vi "SimpelStrategie(SubVI).vi"(4 "toggle":bool, 5 "NextTurn":dbl, 6 "BoolArray":bool[][](array[boolean]), 7 "Array":dbl[][](array[numeric])) -> (0 "toggle 2":bool, 1 "Array 3":bool[][](array[boolean]), 2 "Array 2":u8[][](array[numeric]))   [LabVIEW 2017]
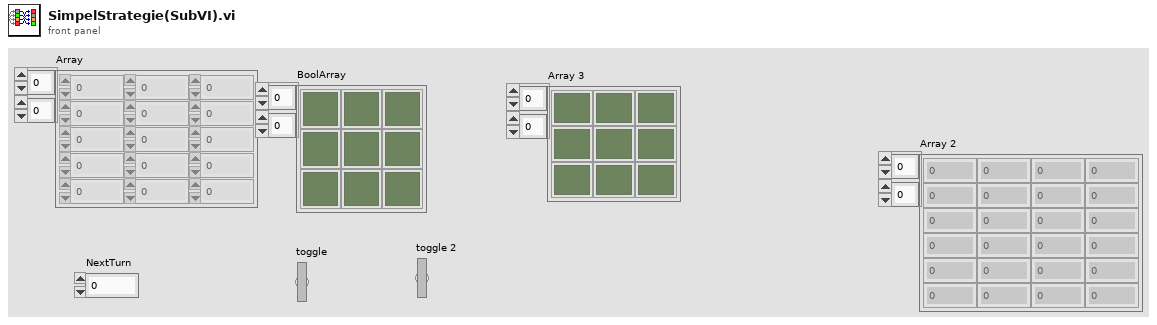
[diagram p1: front panel]
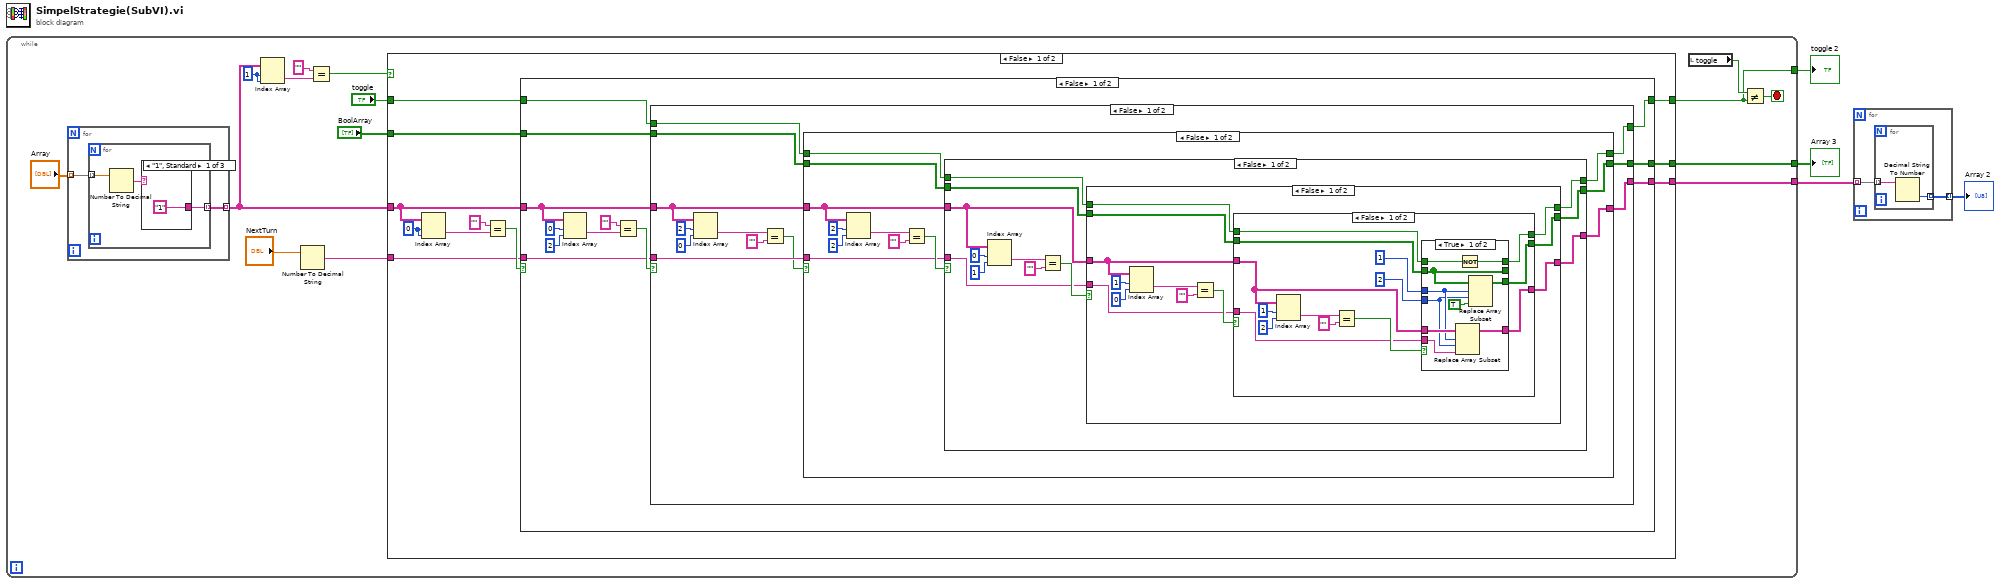
[diagram p0: block diagram]
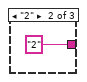
[diagram p2: hidden frame]
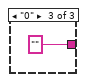
[diagram p3: hidden frame]
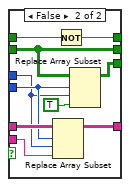
[diagram p4: hidden frame]
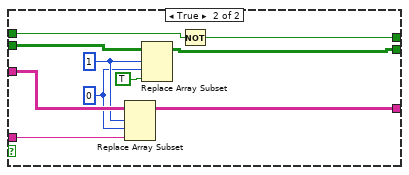
[diagram p5: hidden frame]
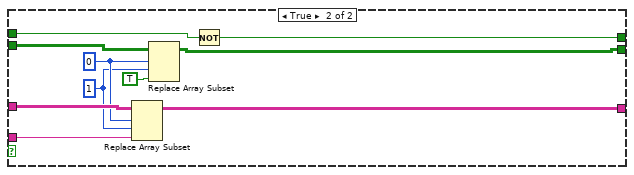
[diagram p6: hidden frame]
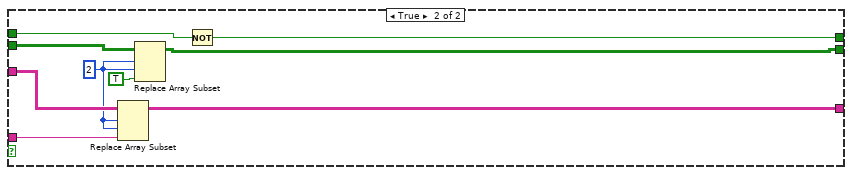
[diagram p7: hidden frame]
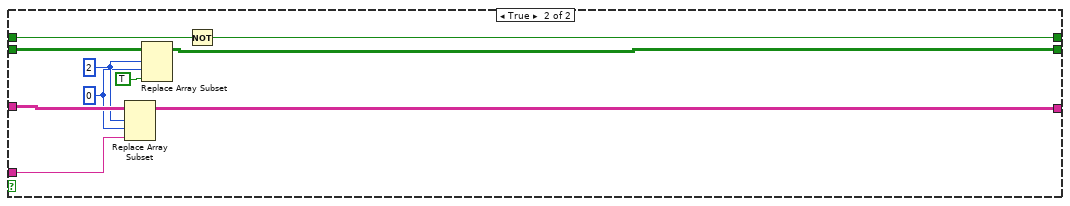
[diagram p8: hidden frame]
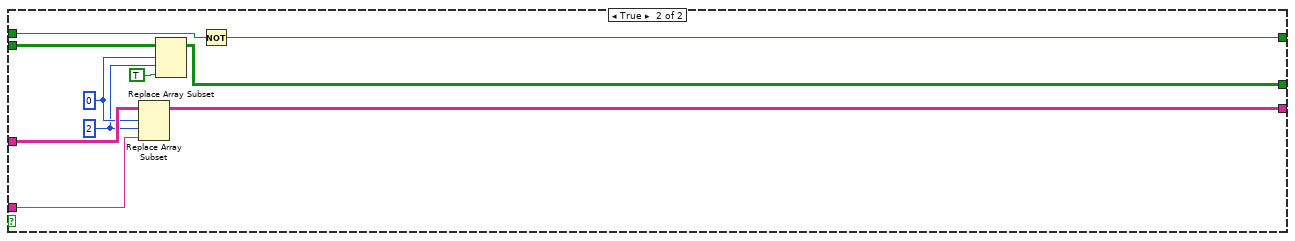
[diagram p9: hidden frame]
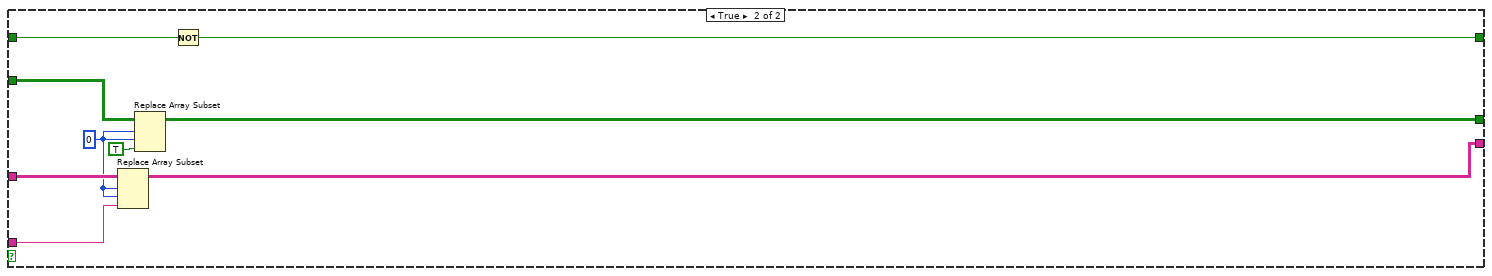
[diagram p10: hidden frame]
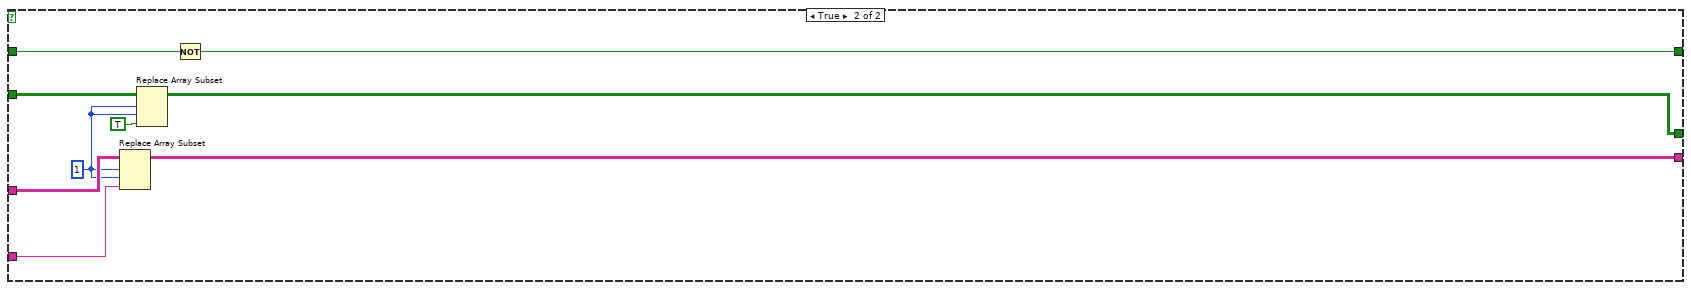
[diagram p11: hidden frame]
diagram:
  n1 = while {
    tunnel: [w10] -> w4
    tunnel: [w13] -> w3
    tunnel: [w12] -> w2
    stop <- w9 stop-if-true
    w19 = 1
    n2 = for {
      tunnel: "Array" -> [w21] mode=indexing
      tunnel: [w20] -> w7 mode=indexing
      n3 = for {
        tunnel: w21 -> [w24] mode=indexing
        tunnel: [w22] -> w20 mode=indexing
        n4 = Number To Decimal String(number=w24) -> (decimal integer string=w23:string)  [unwired: 1 in]
        n5 = case shown="\"1\", Standard" w23 {
          tunnel: ["1" "2" ""] -> w22
          frame "1", Default {
          }
          frame "2" {
          }
          frame "0" {
          }
        }
      }
    }
    n6 = Index Array(array=w7, index (row)=w19, index (col)=w19) -> (element=w15:string)
    n7 = Number To Decimal String(number="NextTurn") -> (decimal integer string=w5:string)  [unwired: 1 in]
    n8 = Equal?(x="", y=w15) -> (x = y?=w18:bool)
    n9 = case shown="False" w18 {
      tunnel: w7 -> [w36 w198]
      tunnel: "BoolArray" -> [w35 w199]
      tunnel: w5 -> [w34 w197]
      tunnel: [w33 w193] -> w12
      tunnel: [w32 w194] -> w13
      tunnel: "toggle" -> [w31 w192]
      tunnel: [w30 w191] -> w10
      frame False {
        w38 = 0
        n10 = Index Array(array=w36, index (row)=w38, index (col)=w38) -> (element=w28:string)
        n11 = Equal?(x="", y=w28) -> (x = y?=w37:bool)
        n12 = case shown="False" w37 {
          tunnel: w36 -> [w47 w190]
          tunnel: w35 -> [w46 w189]
          tunnel: w34 -> [w45 w188]
          tunnel: [w44 w184] -> w33
          tunnel: [w43 w185] -> w32
          tunnel: w31 -> [w42 w183]
          tunnel: [w41 w182] -> w30
          frame False {
            n13 = Index Array(array=w47, index (row)=0, index (col)=2) -> (element=w39:string)
            n14 = Equal?(x="", y=w39) -> (x = y?=w49:bool)
            n15 = case shown="False" w49 {
              tunnel: w47 -> [w58 w181]
              tunnel: w46 -> [w57 w180]
              tunnel: w45 -> [w56 w175]
              tunnel: [w55 w178] -> w44
              tunnel: [w54 w179] -> w43
              tunnel: w42 -> [w52 w173]
              tunnel: [w51 w172] -> w41
              frame False {
                n16 = Index Array(array=w58, index (row)=2, index (col)=0) -> (element=w59:string)
                n17 = Equal?(x=w59, y="") -> (x = y?=w53:bool)
                n18 = case shown="False" w53 {
                  tunnel: w58 -> [w69 w170]
                  tunnel: w57 -> [w68 w171]
                  tunnel: w56 -> [w67 w167]
                  tunnel: [w66 w169] -> w55
                  tunnel: [w65 w168] -> w54
                  tunnel: w52 -> [w64 w163]
                  tunnel: [w63 w162] -> w51
                  frame False {
                    n19 = Index Array(array=w69, index (row)=2, index (col)=2) -> (element=w74:string)
                    n20 = Equal?(x=w74, y="") -> (x = y?=w70:bool)
                    n21 = case shown="False" w70 {
                      tunnel: w69 -> [w81 w159]
                      tunnel: w68 -> [w80 w158]
                      tunnel: w67 -> [w79 w156]
                      tunnel: [w78 w161] -> w66
                      tunnel: [w77 w160] -> w65
                      tunnel: w64 -> [w76 w154]
                      tunnel: [w75 w153] -> w63
                      frame False {
                        n22 = Index Array(array=w81, index (row)=0, index (col)=1) -> (element=w83:string)
                        n23 = Equal?(x=w83, y="") -> (x = y?=w82:bool)
                        n24 = case shown="False" w82 {
                          tunnel: w81 -> [w93 w152]
                          tunnel: w80 -> [w92 w150]
                          tunnel: w79 -> [w91 w146]
                          tunnel: [w90 w151] -> w78
                          tunnel: [w89 w149] -> w77
                          tunnel: w76 -> [w88 w144]
                          tunnel: [w87 w143] -> w75
                          frame False {
                            n25 = Index Array(array=w93, index (row)=1, index (col)=0) -> (element=w98:string)
                            n26 = Equal?(x=w98, y="") -> (x = y?=w94:bool)
                            n27 = case shown="False" w94 {
                              tunnel: w93 -> [w109 w142]
                              tunnel: w92 -> [w108 w141]
                              tunnel: w91 -> [w107 w140]
                              tunnel: [w104 w139] -> w90
                              tunnel: [w103 w138] -> w89
                              tunnel: w88 -> [w100 w134]
                              tunnel: [w99 w133] -> w87
                              frame False {
                                n28 = Index Array(array=w109, index (row)=1, index (col)=2) -> (element=w112:string)
                                n29 = Equal?(x=w112, y="") -> (x = y?=w110:bool)
                                n30 = case shown="True" w110 {
                                tunnel: w109 -> [w122 w132]
                                tunnel: [w120 w130] -> _
                                tunnel: w108 -> [w120 w130]
                                tunnel: w107 -> [w121 w131]
                                tunnel: 1 -> [w119 w123]
                                tunnel: 2 -> [w118 w124]
                                tunnel: [w116 w128] -> w104
                                tunnel: [w115 w127] -> w103
                                tunnel: w100 -> [w114 w126]
                                tunnel: [w113 w125] -> w99
                                frame True {
                                n31 = Replace Array Subset(array=w122, new element=w121, index (row)=w119, index (col)=w118) -> (w116:string[][])
                                n32 = Not(x=w114) -> (.not. x?=w113:bool)
                                n33 = Replace Array Subset(array=w120, new element=TRUE, index (row)=w119, index (col)=w118) -> (w115:bool[][])
                                }
                                frame False {
                                n34 = Replace Array Subset(array=w132, new element=w131, index (row)=w124, index (col)=w123) -> (w128:string[][])
                                n35 = Not(x=w126) -> (.not. x?=w125:bool)
                                n36 = Replace Array Subset(array=w130, new element=TRUE, index (row)=w124, index (col)=w123) -> (w127:bool[][])
                                }
                                }
                              }
                              frame True {
                                w137 = 1
                                w136 = 0
                                n37 = Replace Array Subset(array=w142, new element=w140, index (row)=w137, index (col)=w136) -> (w139:string[][])
                                n38 = Replace Array Subset(array=w141, new element=TRUE, index (row)=w137, index (col)=w136) -> (w138:bool[][])
                                n39 = Not(x=w134) -> (.not. x?=w133:bool)
                              }
                            }
                          }
                          frame True {
                            w148 = 0
                            w147 = 1
                            n40 = Replace Array Subset(array=w152, new element=w146, index (row)=w148, index (col)=w147) -> (w151:string[][])
                            n41 = Replace Array Subset(array=w150, new element=TRUE, index (row)=w148, index (col)=w147) -> (w149:bool[][])
                            n42 = Not(x=w144) -> (.not. x?=w143:bool)
                          }
                        }
                      }
                      frame True {
                        w155 = 2
                        n43 = Replace Array Subset(array=w159, new element=w156, index (row)=w155, index (col)=w155) -> (w161:string[][])
                        n44 = Replace Array Subset(array=w158, new element=TRUE, index (row)=w155, index (col)=w155) -> (w160:bool[][])
                        n45 = Not(x=w154) -> (.not. x?=w153:bool)
                      }
                    }
                  }
                  frame True {
                    w165 = 2
                    w164 = 0
                    n46 = Replace Array Subset(array=w170, new element=w167, index (row)=w165, index (col)=w164) -> (w169:string[][])
                    n47 = Replace Array Subset(array=w171, new element=TRUE, index (row)=w165, index (col)=w164) -> (w168:bool[][])
                    n48 = Not(x=w163) -> (.not. x?=w162:bool)
                  }
                }
              }
              frame True {
                w177 = 0
                w176 = 2
                n49 = Replace Array Subset(array=w181, new element=w175, index (row)=w177, index (col)=w176) -> (w178:string[][])
                n50 = Replace Array Subset(array=w180, new element=TRUE, index (row)=w177, index (col)=w176) -> (w179:bool[][])
                n51 = Not(x=w173) -> (.not. x?=w172:bool)
              }
            }
          }
          frame True {
            w187 = 0
            n52 = Replace Array Subset(array=w190, new element=w188, index (row)=w187, index (col)=w187) -> (w184:string[][])
            n53 = Replace Array Subset(array=w189, new element=TRUE, index (row)=w187, index (col)=w187) -> (w185:bool[][])
            n54 = Not(x=w183) -> (.not. x?=w182:bool)
          }
        }
      }
      frame True {
        w196 = 1
        n55 = Replace Array Subset(array=w198, new element=w197, index (row)=w196, index (col)=w196) -> (w193:string[][])
        n56 = Replace Array Subset(array=w199, new element=TRUE, index (row)=w196, index (col)=w196) -> (w194:bool[][])
        n57 = Not(x=w192) -> (.not. x?=w191:bool)
      }
    }
    n58 = local read "toggle"() -> (w11:bool)
    n59 = Not Equal?(x=w11, y=w10) -> (x != y?=w9:bool)
  }
  "toggle 2" <- w4
  "Array 3" <- w3
  n60 = for {
    tunnel: w2 -> [w201] mode=indexing
    tunnel: [w200] -> w1 mode=indexing
    n61 = for {
      tunnel: w201 -> [w203] mode=indexing
      tunnel: [w202] -> w200 mode=indexing
      n62 = Decimal String To Number(string=w203) -> (number=w202:i32)  [unwired: 2 in, 1 out]
    }
  }
  "Array 2" <- w1
